vi "Toolkit Error Handling - Trim Call Chain at First API VI.vi"(8 "error in (no error)":errorcluster, 9 "API VI List":string[](array[string]), 10 "call chain":string[](array[string])) -> (0 "error out":errorcluster, 2 "trimmed call chain":string[](array[string]))   [LabVIEW 2013]
doc: "Trims the call chain, removing everything below the Toolkit API VIs"
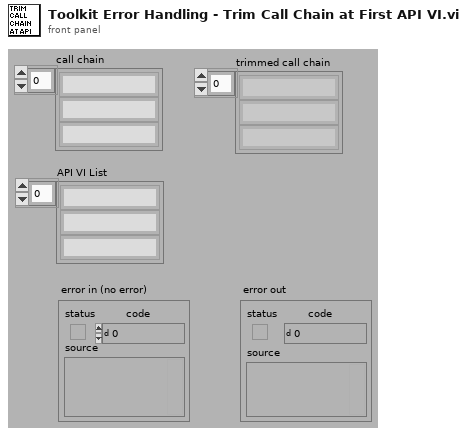
[diagram p1: front panel]
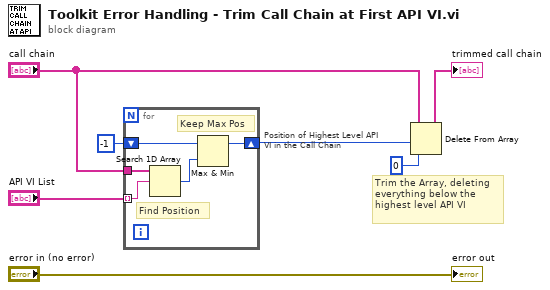
[diagram p0: block diagram]
diagram:
  # "Trim the Array, deleting everything below the highest level API VI"
  # "Position of Highest Level API VI in the Call Chain"
  n1 = for {
    tunnel: "API VI List" -> [w11] mode=indexing
    tunnel: "call chain" -> [w12]
    shift-right: [w10] -> w2
    shift-left: -1 ("index of element") -> [w8]
    # "Find Position"
    # "Keep Max Pos"
    n2 = Search 1D Array(1D array=w12, element=w11) -> (index of element=w9:i32)  [unwired: 1 in]
    n3 = Max & Min(x=w8, y=w9) -> (max(x,y)=w10:i32)  [unwired: 1 out]
  }
  n4 = Delete From Array(array="call chain", length=w2, index=0) -> (array with subset deleted=→"trimmed call chain":string[])  [unwired: 1 out]
  "error out" <- "error in (no error)"
